vi "Read limits csv.vi"(8 "error in (no error)":errorcluster, 11 "file path":path) -> (0 "error out":errorcluster, 2 "Limits_data":string[][](array[string]), 3 "Dup file path":path)   [LabVIEW 2018]
uses:
  <vilib>/Utility/file.llb/Read Delimited Spreadsheet (string).vi
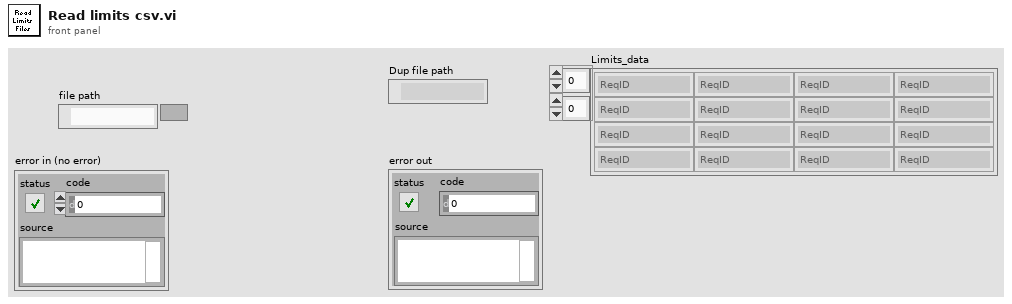
[diagram p1: front panel]
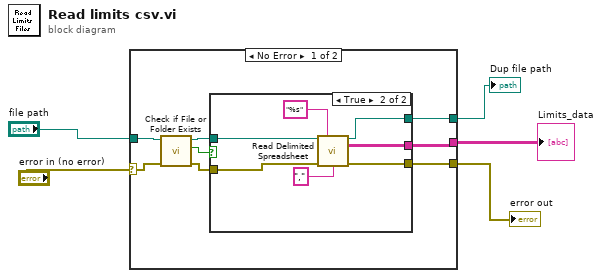
[diagram p0: block diagram]
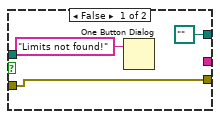
[diagram p2: hidden frame]
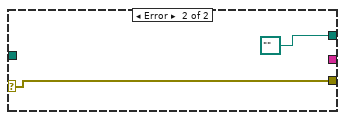
[diagram p3: hidden frame]
diagram:
  n1 = case shown="No Error" "error in (no error)" {
    selector: "error in (no error)" -> [w10 w25]
    tunnel: [w13 w25] -> w4
    tunnel: "file path" -> [w12 _]
    tunnel: [w7 path "" ("new file path (Not A Path if cancelled)")] -> w2
    tunnel: [w6 _] -> w1
    frame No Error {
      n2 = call <vilib>:"Check if File or Folder Exists.vi"("error in (no error)"=w10, "path"=w12) -> ("error out"=w9:errorcluster, "file or folder exists?"=w8:bool, "dup path"=w11:path)  [unwired: 7 in]
      n3 = case shown="True" w8 {
        tunnel: w9 -> [w16 w23]
        tunnel: [w16 w22] -> w13
        tunnel: w11 -> [_ w21]
        tunnel: [path "" ("new file path (Not A Path if cancelled)") w18] -> w7
        tunnel: [_ w17] -> w6
        frame False {
          n4 = One Button Dialog(message="Limits not found!") -> ()  [unwired: 1 in, 1 out]
        }
        frame True {
          n5 = call-poly <vilib>:"Read Delimited Spreadsheet.vi"("file path (dialog if empty)"=w21, "format (%s)"="%s", "error in (no error)"=w23, "delimiter (\\t)"="," ("delimiter (\\t)")) -> ("new file path (Not A Path if cancelled)"=w18:path, "all rows"=w17:string[][], "error out"=w22:errorcluster)  [unwired: 6 in, 3 out]
        }
      }
    }
    frame Error {
    }
  }
  "error out" <- w4
  "Dup file path" <- w2
  "Limits_data" <- w1
